vi "EVS Main Dev.vi"() -> ()   [LabVIEW 2009]
uses:
  <vilib>/userDefined/High Color/IMAQdx.ctl
  UDP Lib/UDP Network Location.ctl
  <vilib>/vision/driver/IMAQdx.llb/IMAQdx Acquisition Mode.ctl
  <vilib>/Platform/TimedLoop/XDataNode/XDataNode.xnode
  <vilib>/Platform/TimedLoop/XDataNode/loadlvalarms.vi
  <vilib>/Platform/TimedLoop/XDataNode/timing_clust.ctl
  <vilib>/Platform/TimedLoop/XDataNode/nitl_modes.ctl
  <vilib>/Platform/TimedLoop/XDataNode/wakeup.ctl
  <vilib>/vision/driver/NI_Vision_Acquisition_Software.lvlib
  <vilib>/Platform/TimedLoop/XDataNode/XDNodeRunTimeDep.lvlib
panel:
  out "Extracted 2":T1(plugin-control) caption="Extracted"
  in  "IMAQdx Session Center":T2="rcam" caption="Center Session"
  out "Original":T1(plugin-control)
  out "Extracted":T1(plugin-control)
  out "Ramp?":bool
  out "Iteration Duration":i64
  out "Number of ramp regions (left)":i32
  out "Number of ramp regions (right)":i32
  out "Sick array":u16[](array[numeric])
  in  "stop":bool
  out "HB":bool
  in  "IMAQdx Session Left":T2="lcam" caption="Left Session"
  in  "IMAQdx Session Right":T2="rcam" caption="Right Session"
  # "0: Original\n1: Extracted\n2: Masked"
  # "0: Old line extraction\n1: Solid white line (ramp)\n2: LPF"
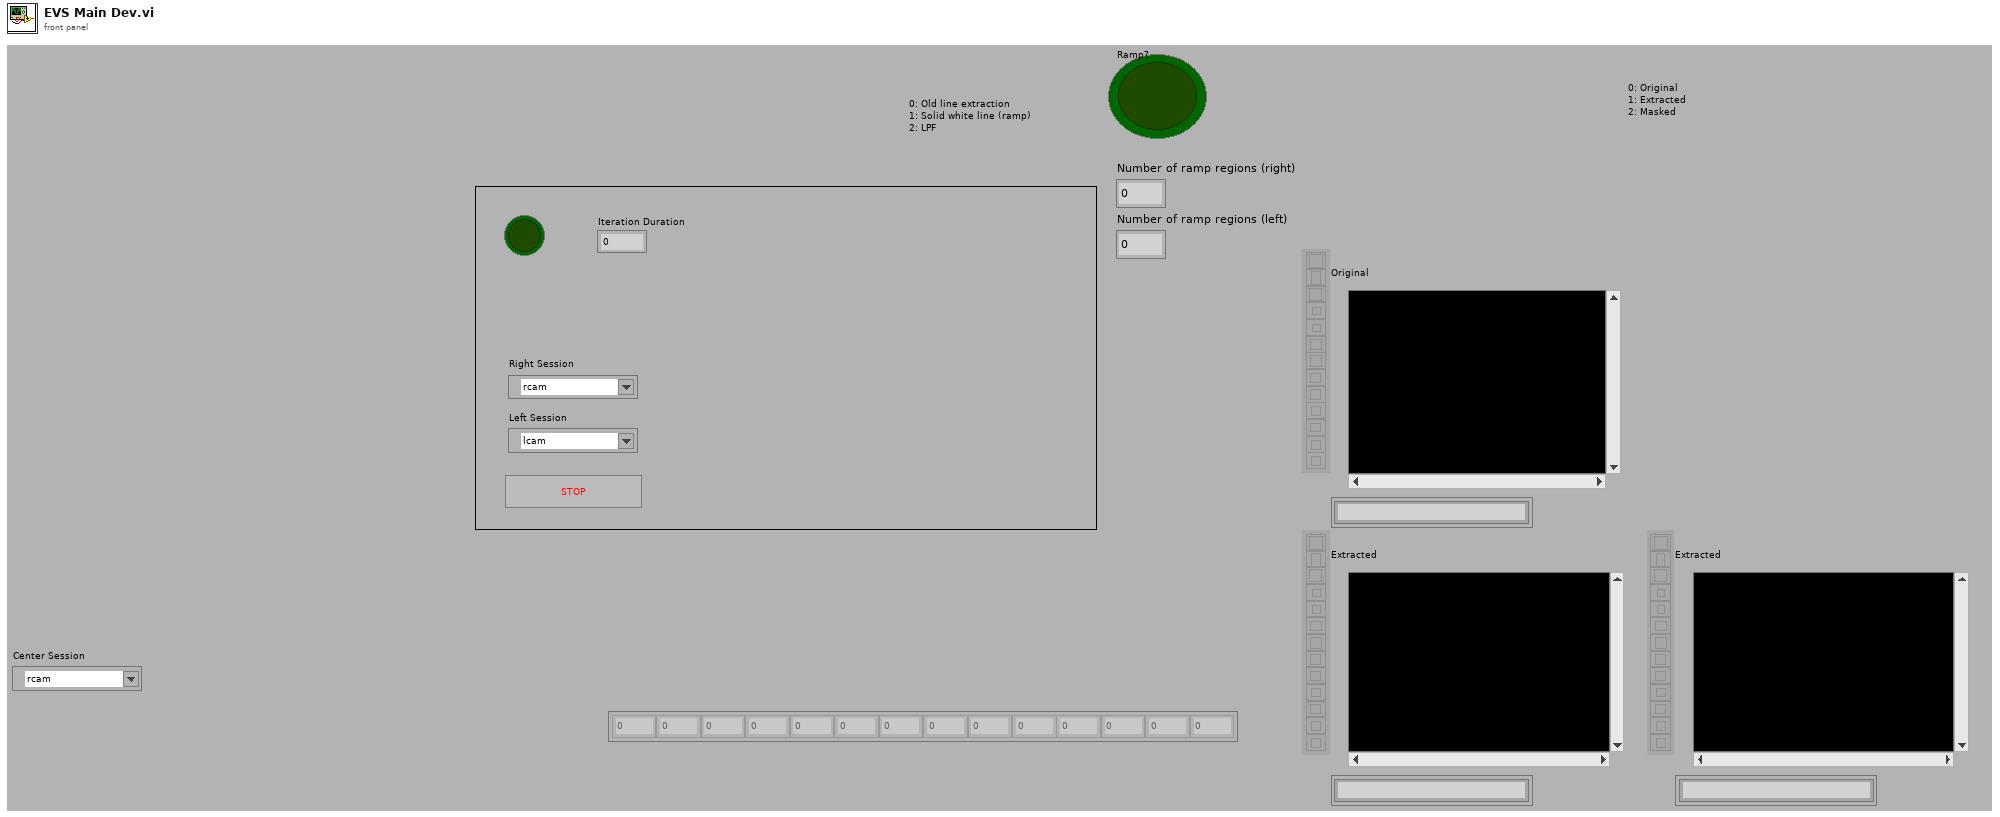
[diagram p1: front panel]
types:
  T1 = typedef "IMAQ Image.ctl" = refnum<image>
  T2 = typedef "IMAQdx.ctl" = refnum<k21>
  T3 = cluster{"Sick array":u16[], "Camera init":bool, "Objects Array":cluster{"X Coord":dbl[], "Y Coord":dbl[]}[]}
  T4 = typedef "NI_Vision_Acquisition_Software.lvlib/IMAQdx Acquisition Mode.ctl" = enum32{"One Shot", "Continuous"}
  T5 = typedef "XDNodeRunTimeDep.lvlib/timing_clust.ctl" = cluster{"Expected End [f-1]":u64, "Actual End [f-1]":u64, "Finished Late? [f-1]":bool, "Expected End [i-1]":u64, "Actual End [i-1]":u64, "Finished Late? [i-1]":bool, "Expected Start [i]":u64, "Actual Start [i]":u64, "Expected Start [f]":u64, "Actual Start [f]":u64, "Source Name":string, "Structure Name":string, "Period":i64, "Deadline":i64, "Offset":i64, "Start":i64, "Priority":i32, "Timeout":i32, "Mode":T6, "Wakeup Reason":T7, "Error":errorcluster, "Source Type":string, "Secondary Source Type":string, "Global End Time":u64, "Global Start Time":u64, "Frame Duration":u64, "Iteration Duration":u64, "Assigned CPU":i32, "I/O Scan Engine Mode":u32}
  T6 = typedef "XDNodeRunTimeDep.lvlib/nitl_modes.ctl" = enum32{"No Change", "Process missed periods, maintain original phase", "Discard missed periods, maintain original phase", "Process missed periods, ignore original phase", "Discard missed periods, ignore original phase"}
  T7 = typedef "XDNodeRunTimeDep.lvlib/wakeup.ctl" = enum32{"Normal", "Aborted", "Asynchronous wakeup", "Timing source error", "Timed loop error", "Timeout"}
  T8 = typedef "UDP Network Location.ctl" = cluster{"IP Address":string, "Port":u16}
  T9 = typedef "UDP Base.ctl" = cluster{"UDP Session":refnum<k16>, "UDP Socket Params":T10}
  T10 = typedef "UDP Socket Params.ctl" = cluster{"Local Port":u16, "Read Timeout":i32, "Write Timeout":i32}
  T11 = typedef "Image Type" = u32
  T12 = cluster{"Sick array":u16[], "Camera init":bool, "Objects Array":cluster{"X Coord":dbl[], "Y Coord":dbl[]}[], bool}
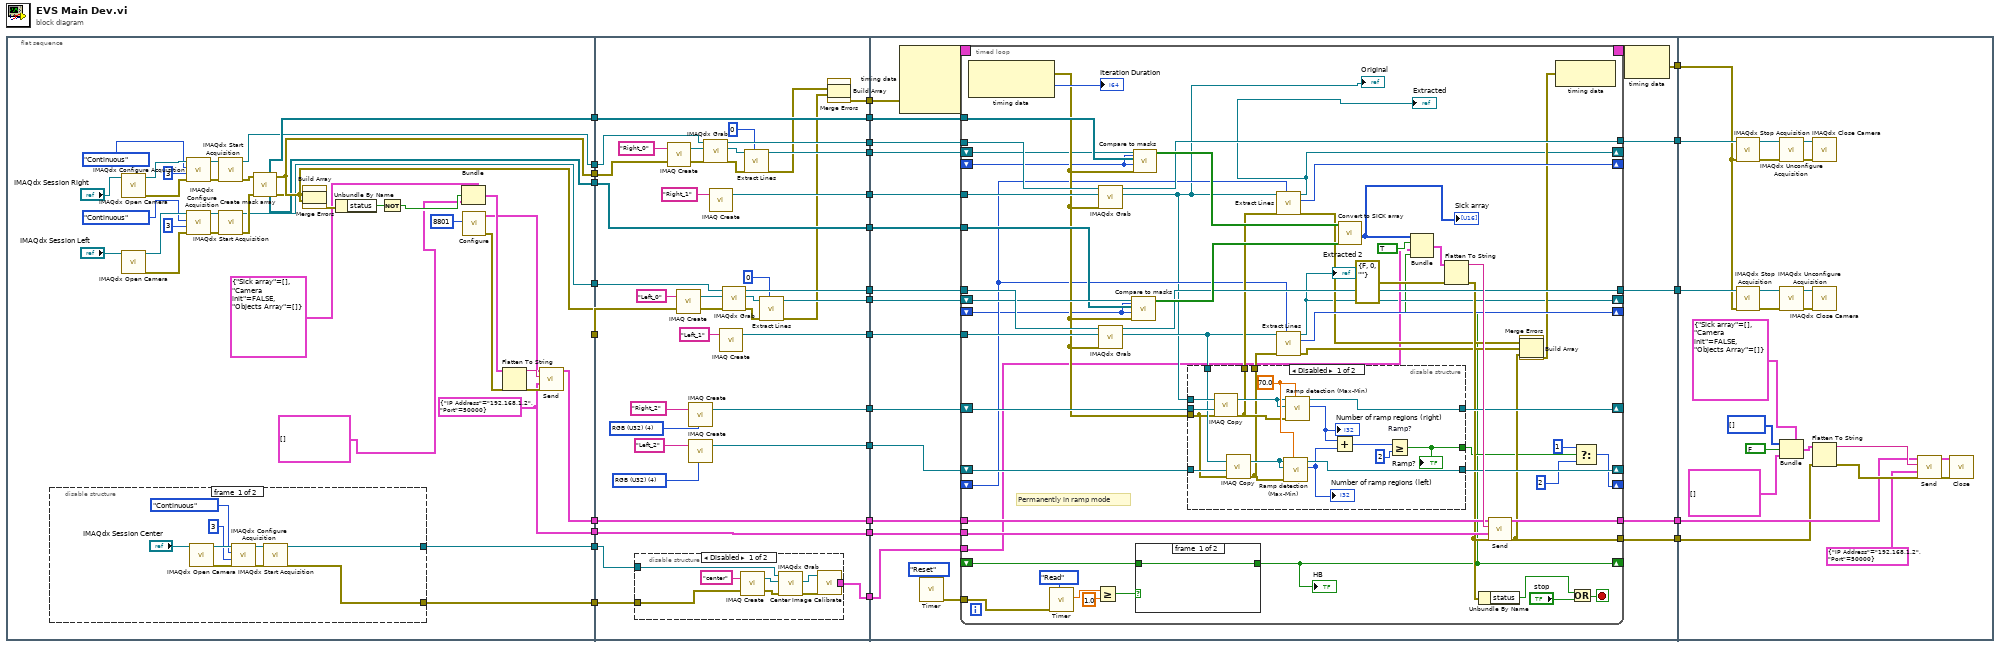
[diagram p0: block diagram]
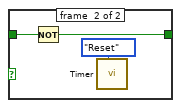
[diagram p4: hidden frame]
diagram:
  n1 = flat-sequence {
    tunnel: [w47] -> w29
    tunnel: [w46] -> w28
    tunnel: [w45] -> w27
    tunnel: [w35] -> w26
    tunnel: [w44] -> w19
    tunnel: [w43] -> w17
    tunnel: [w42] -> w16
    tunnel: [w39] -> w8
    tunnel: [w34] -> w3
    tunnel: [w33] -> w2
    tunnel: w29 -> [w109]
    tunnel: w28 -> [w108]
    tunnel: w27 -> [w105]
    tunnel: w26 -> [w104]
    tunnel: [w103] -> w25
    tunnel: [w100] -> w24
    tunnel: [w99] -> w23
    tunnel: [w98] -> w22
    tunnel: [w97] -> w21
    tunnel: [w96] -> w20
    tunnel: w19 -> [w95]
    tunnel: [w95] -> w18
    tunnel: w17 -> [w94]
    tunnel: w16 -> [w93]
    tunnel: [w94] -> w15
    tunnel: [w93] -> w14
    tunnel: [w92] -> w9
    tunnel: w8 -> [w92]
    tunnel: [w89] -> w7
    tunnel: [w88] -> w6
    tunnel: [w85] -> w5
    tunnel: w3 -> [w80]
    tunnel: w2 -> [w79]
    tunnel: [w78] -> w1
    tunnel: w25 -> [w137]
    tunnel: w24 -> [w136]
    tunnel: w23 -> [w148]
    tunnel: w22 -> [w147]
    tunnel: w21 -> [w146]
    tunnel: w20 -> [w145]
    tunnel: w18 -> [w144]
    tunnel: w15 -> [w143]
    tunnel: w14 -> [w142]
    tunnel: [w141] -> w13
    tunnel: [w140] -> w12
    tunnel: [w139] -> w11
    tunnel: [w138] -> w10
    tunnel: w9 -> [w135]
    tunnel: w7 -> [w132]
    tunnel: w6 -> [w131]
    tunnel: w5 -> [w130]
    tunnel: [w129] -> w4
    tunnel: w1 -> [w128]
    tunnel: w13 -> [w253]
    tunnel: w12 -> [w252]
    tunnel: w11 -> [w248]
    tunnel: w10 -> [w247]
    tunnel: w4 -> [w241]
    frame #0 {
      w39 = T8 {"IP Address"="192.168.1.2", "Port"=50000} ("cRIO Network Location")
      n2 = disable-structure shown="Enabled" {
        disable-tunnel: [w69 _] -> w34
        disable-tunnel: [w68 _] -> w33
        frame #0 {
          n3 = call <vilib>:"IMAQdx Open Camera.vi"("Session In"="IMAQdx Session Center") -> ("error out"=w75:errorcluster, "Session Out"=w74:T2)  [unwired: 2 in, 7 out]
          n4 = call <vilib>:"IMAQdx Configure Acquisition.vi"("error in"=w75, "Number of Buffers"=u32 3, "Continuous?"=IMAQdx_Acquisition_Mode."Continuous", "Session In"=w74) -> ("error out"=w76:errorcluster, "Session Out"=w73:T2)  [unwired: 1 in, 5 out]
          n5 = call <vilib>:"IMAQdx Start Acquisition.vi"("error in"=w76, "Session In"=w73) -> ("error out"=w68:errorcluster, "Session Out"=w69:T2)  [unwired: 8 out]
        }
        frame #1 {
        }
      }
      n6 = call <vilib>:"IMAQdx Open Camera.vi"("Session In"="IMAQdx Session Right") -> ("error out"=w66:errorcluster, "Session Out"=w65:T2)  [unwired: 2 in, 7 out]
      n7 = call <vilib>:"IMAQdx Open Camera.vi"("Session In"="IMAQdx Session Left") -> ("error out"=w60:errorcluster, "Session Out"=w61:T2)  [unwired: 2 in, 7 out]
      n8 = call <vilib>:"IMAQdx Configure Acquisition.vi"("error in"=w66, "Number of Buffers"=u32 3, "Continuous?"=IMAQdx_Acquisition_Mode."Continuous", "Session In"=w65) -> ("error out"=w67:errorcluster, "Session Out"=w64:T2)  [unwired: 1 in, 5 out]
      n9 = call <vilib>:"IMAQdx Configure Acquisition.vi"("error in"=w60, "Number of Buffers"=u32 3, "Continuous?"=IMAQdx_Acquisition_Mode."Continuous", "Session In"=w61) -> ("error out"=w59:errorcluster, "Session Out"=w62:T2)  [unwired: 1 in, 5 out]
      n10 = call <vilib>:"IMAQdx Start Acquisition.vi"("error in"=w67, "Session In"=w64) -> ("error out"=w53:errorcluster, "Session Out"=w35:T2)  [unwired: 8 out]
      n11 = call <vilib>:"IMAQdx Start Acquisition.vi"("error in"=w59, "Session In"=w62) -> ("error out"=w52:errorcluster, "Session Out"=w45:T2)  [unwired: 8 out]
      n12 = call "Create mask array.vi"("Left error in"=w52, "Right Error in"=w53) -> ("Left error out"=w46:errorcluster, "Right error out"=w47:errorcluster, "Left Cam Masks"=w42:T1[], "Right Cam Masks"=w43:T1[])  [unwired: 6 in]
      n13 = Build Array(w47, w46) -> (w32:errorcluster[])
      n14 = call <vilib>:"Merge Errors.vi"("error array in"=w32) -> ("error out"=w40:errorcluster)  [unwired: 6 in]
      n15 = Unbundle By Name(w40) -> ("status"=w51:bool)
      n16 = Not(x=w51) -> (.not. x?=w41:bool)
      n17 = Bundle(cluster=T3 {"Sick array"=[], "Camera init"=FALSE, "Objects Array"=[]}, "Camera init"=w41, "Objects Array"=cluster{"X Coord":dbl[], "Y Coord":dbl[]}[] []) -> (w50:T3)  [unwired: 1 in]
      n18 = call "Configure.vi"("Local Port"=u16 8801) -> ("error out"=w36:errorcluster, "UDP Base out"=w37:T9)  [unwired: 9 in]
      n19 = Flatten To String(anything=w50, error in (no error)=w36) -> (data string=w49:string, error out=w48:errorcluster)  [unwired: 2 in, 1 out]
      n20 = call "Send.vi"("error in (no error)"=w48, "Destination Location"=w39, "Send Data"=w49, "UDP Base in"=w37) -> ("UDP Base out"=w44:T9)  [unwired: 5 in, 2 out]
    }
    frame #1 {
      w83 = T11 4 items=["Grayscale (U8)", "Grayscale (I16)", "Grayscale (SGL)", "Complex (CSG)", "RGB (U32)", "HSL (U32)", "RGB (U64)", "Grayscale (U16)"] ("Image Type")
      w84 = T11 4 items=["Grayscale (U8)", "Grayscale (I16)", "Grayscale (SGL)", "Complex (CSG)", "RGB (U32)", "HSL (U32)", "RGB (U64)", "Grayscale (U16)"] ("Image Type")
      n21 = disable-structure shown="Disabled" {
        disable-tunnel: w80 -> [w120 _]
        disable-tunnel: w79 -> [w119 _]
        disable-tunnel: [w118 _] -> w78
        frame #0 {
          n22 = call "IMAQ Create"("Image Name"="center", "error in (no error)"=w119) -> ("New Image"=w121:T1, "error out"=w122:errorcluster)  [unwired: 3 in]
          n23 = call <vilib>:"IMAQdx Grab.vi"("error in"=w122, "Image In"=w121, "Session In"=w120) -> ("error out"=w125:errorcluster, "Image Out"=w124:T1)  [unwired: 5 in, 2 out]
          n24 = call "Center Image Calibrate.vi"("error in"=w125, "Image In"=w124) -> ("Objects Array"=w118:cluster{"X Coord":dbl[], "Y Coord":dbl[]}[])  [unwired: 1 in, 2 out]
        }
        frame #1 {
        }
      }
      n25 = call "IMAQ Create"("Image Name"="Right_0", "error in (no error)"=w109) -> ("New Image"=w111:T1, "error out"=w110:errorcluster)  [unwired: 3 in]
      n26 = call "IMAQ Create"("Image Name"="Left_0", "error in (no error)"=w108) -> ("New Image"=w113:T1, "error out"=w112:errorcluster)  [unwired: 3 in]
      n27 = call "IMAQ Create"("Image Name"="Right_2", "Image Type"=w84) -> ("New Image"=w89:T1)  [unwired: 3 in, 1 out]
      n28 = call "IMAQ Create"("Image Name"="Left_2", "Image Type"=w83) -> ("New Image"=w88:T1)  [unwired: 3 in, 1 out]
      n29 = call <vilib>:"IMAQdx Grab.vi"("error in"=w110, "Image In"=w111, "Session In"=w104) -> ("error out"=w117:errorcluster, "Image Out"=w114:T1, "Session Out"=w99:T2)  [unwired: 5 in, 1 out]
      n30 = call "IMAQ Create"("Image Name"="Right_1") -> ("New Image"=w103:T1)  [unwired: 4 in, 1 out]
      n31 = call "IMAQ Create"("Image Name"="Left_1") -> ("New Image"=w100:T1)  [unwired: 4 in, 1 out]
      n32 = call <vilib>:"IMAQdx Grab.vi"("error in"=w112, "Image In"=w113, "Session In"=w105) -> ("error out"=w116:errorcluster, "Image Out"=w115:T1, "Session Out"=w98:T2)  [unwired: 5 in, 1 out]
      n33 = call "Extract Lines.vi"("Extraction mode"=0, "error in (no error)"=w117, "Image Src"=w114) -> ("error out"=w87:errorcluster, "Image Out"=w97:T1)  [unwired: 6 in, 1 out]
      n34 = call "Extract Lines.vi"("Extraction mode"=0, "error in (no error)"=w116, "Image Src"=w115) -> ("error out"=w86:errorcluster, "Image Out"=w96:T1)  [unwired: 6 in, 1 out]
      n35 = Build Array(w87, w86) -> (w77:errorcluster[])
      n36 = call <vilib>:"Merge Errors.vi"("error array in"=w77) -> ("error out"=w85:errorcluster)  [unwired: 6 in]
    }
    frame #2 {
      n37 = node-c288(w130) -> (w134:T5)  [unwired: 3 in]
      n38 = call "Timer.vi"("Cmd"=enum16{"Reset", "Read"}."Reset") -> ("error out"=w126:errorcluster)  [unwired: 9 in, 1 out]
      n39 = timed-loop {
        tunnel: w148 -> [w206]
        tunnel: w147 -> [w205]
        shift-right: [w161] -> _
        shift-left: w146 -> [w162]
        shift-right: [w155] -> _
        shift-left: w145 -> [w204]
        shift-right: [w179] -> _
        shift-left: _ -> [w158]
        shift-right: [w180] -> _
        shift-left: _ -> [w159]
        tunnel: w144 -> [w200]
        tunnel: [w199] -> w139
        tunnel: [w173] -> w138
        tunnel: w143 -> [w198]
        tunnel: w142 -> [w197]
        tunnel: [w196] -> w140
        tunnel: [w195] -> w141
        tunnel: w137 -> [w194]
        tunnel: w136 -> [w193]
        tunnel: w135 -> [w189]
        shift-right: [w149] -> _
        shift-left: _ -> [w188]
        timing: w134 -> [_]
        timing-out: [_] -> w133
        shift-right: [w186] -> _
        shift-left: w132 -> [w178]
        shift-right: [w185] -> _
        shift-left: w131 -> [w177]
        shift-right: [w164] -> _
        shift-left: _ -> [w168]
        tunnel: w128 -> [w157]
        tunnel: w126 -> [w153]
        stop <- w184 stop-if-true
        # "Permanently in ramp mode"
        n40 = node-c288() -> (w176:errorcluster, →"Iteration Duration":i64)  [unwired: 1 in]
        n41 = call "Timer.vi"("Cmd"=enum16{"Reset", "Read"}."Read", "error in (no error)"=w153) -> ("Elapsed Time"=w152:dbl)  [unwired: 8 in, 1 out]
        n42 = Greater Or Equal?(x=w152, y=1.0) -> (x >= y?=w150:bool)
        n43 = call <vilib>:"IMAQdx Grab.vi"("error in"=w176, "Image In"=w194, "Session In"=w206) -> ("Image Out"=w160:T1, "Session Out"=w196:T2)  [unwired: 5 in, 2 out]
        "Original" <- w160
        n44 = call <vilib>:"IMAQdx Grab.vi"("error in"=w176, "Image In"=w193, "Session In"=w205) -> ("Image Out"=w163:T1, "Session Out"=w195:T2)  [unwired: 5 in, 2 out]
        n45 = call "Compare to masks.vi"("Number of Particles1"=w158, "error in (no error)"=w176, "Number of Particles"=w158, "Mask array"=w197, "Image Src"=w204) -> ("Marked Regions"=w202:bool[])  [unwired: 5 in, 1 out]
        n46 = call "Compare to masks.vi"("Number of Particles1"=w159, "error in (no error)"=w176, "Number of Particles"=w159, "Mask array"=w198, "Image Src"=w162) -> ("Marked Regions"=w203:bool[])  [unwired: 5 in, 1 out]
        n47 = case shown="True" w150 {
          tunnel: [w207 w210] -> w149
          tunnel: w188 -> [w207 w209]
          frame #0 {
          }
          frame #1 {
            n48 = Not(x=w209) -> (.not. x?=w210:bool)
            n49 = call "Timer.vi"("Cmd"=enum16{"Reset", "Read"}."Reset") -> ()  [unwired: 9 in, 2 out]
          }
        }
        "HB" <- w149
        n50 = disable-structure shown="Disabled" {
          disable-tunnel: [w227 _] -> w186
          disable-tunnel: [w226 _] -> w185
          disable-tunnel: [w220 _] -> w167
          disable-tunnel: w178 -> [w219 _]
          disable-tunnel: w160 -> [w218 _]
          disable-tunnel: w163 -> [w217 _]
          disable-tunnel: w177 -> [w216 _]
          disable-tunnel: w176 -> [w215 _]
          disable-tunnel: [w212 _] -> w170
          disable-tunnel: [w211 _] -> w169
          frame #0 {
            w225 = sgl 70.0 ("Tolerance")
            n51 = call "IMAQ Copy"("error in (no error)"=w215, "Image Dst"=w219, "Image Src"=w218) -> ("error out"=w212:errorcluster, "Image Dst Out"=w214:T1)  [unwired: 3 in]
            n52 = call "IMAQ Copy"("error in (no error)"=w215, "Image Dst"=w216, "Image Src"=w217) -> ("error out"=w211:errorcluster, "Image Dst Out"=w213:T1)  [unwired: 3 in]
            n53 = call "Ramp detection (Max-Min).vi"("Tolerance"=w225, "error in (no error)"=w211, "Image Dst"=w213, "Image Src"=w213) -> ("Number of ramp regions"=w223:i32, "Image Out"=w226:T1)  [unwired: 5 in, 1 out]
            "Number of ramp regions (left)" <- w223
            n54 = call "Ramp detection (Max-Min).vi"("Tolerance"=w225, "error in (no error)"=w212, "Image Dst"=w214, "Image Src"=w214) -> ("Number of ramp regions"=w224:i32, "Image Out"=w227:T1)  [unwired: 5 in, 1 out]
            "Number of ramp regions (right)" <- w224
            n55 = Add(x=w224, y=w223) -> (x+y=w222:i32)
            n56 = Greater Or Equal? "Ramp?"(x=w222, y=2) -> (x >= y?=w220:bool)
            "Ramp?" <- w220
          }
          frame #1 {
          }
        }
        n57 = call "Extract Lines.vi"("Extraction mode"=w168, "error in (no error)"=w170, "Image Src"=w160) -> ("error out"=w172:errorcluster, "Number of Particles1"=w180:i32, "Image Out"=w161:T1)  [unwired: 6 in]
        "Extracted" <- w161
        n58 = call "Extract Lines.vi"("Extraction mode"=w168, "error in (no error)"=w169, "Image Src"=w163) -> ("error out"=w171:errorcluster, "Number of Particles1"=w179:i32, "Image Out"=w155:T1)  [unwired: 6 in]
        "Extracted 2" <- w155
        n59 = call "Convert to SICK array.vi"("Left Regions"=w202, "Right Regions"=w203) -> ("Sick array"=w175:u16[])  [unwired: 9 in]
        "Sick array" <- w175
        n60 = Bundle("Sick array"=w175, "Camera init"=TRUE, "Objects Array"=w157, w149) -> (w190:T12)  [unwired: 1 in]
        n61 = Flatten To String(anything=w190, error in (no error)=errorcluster {"status"=FALSE, "code"=0, "source"=""} ("error out")) -> (data string=w201:string, error out=w181:errorcluster)  [unwired: 2 in, 1 out]
        n62 = Unbundle By Name(w181) -> ("status"=w192:bool)
        n63 = call "Send.vi"("error in (no error)"=w181, "Destination Location"=w189, "Send Data"=w201, "UDP Base in"=w200) -> ("error out"=w173:errorcluster, "UDP Base out"=w199:T9)  [unwired: 5 in, 1 out]
        n64 = Build Array(w172, w171, w173) -> (w156:errorcluster[])
        n65 = call <vilib>:"Merge Errors.vi"("error array in"=w156) -> ("error out"=w174:errorcluster)  [unwired: 6 in]
        n66 = node-c288(w174) -> ()  [unwired: 1 out]
        n67 = Or(x=w192, y="stop") -> (x .or. y?=w184:bool)
        n68 = Select(t=1, s=w167, f=2 ("Extraction mode")) -> (s? t:f=w164:i32)
      }
      n69 = node-c288(w133) -> (w129:errorcluster)
    }
    frame #3 {
      n70 = call <vilib>:"IMAQdx Stop Acquisition.vi"("error in"=w241, "Session In"=w252) -> ("error out"=w259:errorcluster, "Session Out"=w258:T2)  [unwired: 8 out]
      n71 = call <vilib>:"IMAQdx Stop Acquisition.vi"("error in"=w241, "Session In"=w253) -> ("error out"=w255:errorcluster, "Session Out"=w254:T2)  [unwired: 8 out]
      n72 = call <vilib>:"IMAQdx Unconfigure Acquisition.vi"("error in"=w259, "Session In"=w258) -> ("error out"=w260:errorcluster, "Session Out"=w261:T2)  [unwired: 8 out]
      n73 = call <vilib>:"IMAQdx Unconfigure Acquisition.vi"("error in"=w255, "Session In"=w254) -> ("error out"=w256:errorcluster, "Session Out"=w257:T2)  [unwired: 8 out]
      n74 = Bundle(cluster=T3 {"Sick array"=[], "Camera init"=FALSE, "Objects Array"=[]}, "Sick array"=u16[] [] ("Camera SICK"), "Camera init"=FALSE, "Objects Array"=cluster{"X Coord":dbl[], "Y Coord":dbl[]}[] []) -> (w243:T3)
      n75 = call <vilib>:"IMAQdx Close Camera.vi"("error in"=w260, "Session In"=w261) -> ()  [unwired: 10 out]
      n76 = call <vilib>:"IMAQdx Close Camera.vi"("error in"=w256, "Session In"=w257) -> ()  [unwired: 10 out]
      n77 = Flatten To String(anything=w243, error in (no error)=w247) -> (data string=w251:string, error out=w250:errorcluster)  [unwired: 2 in, 1 out]
      n78 = call "Send.vi"("error in (no error)"=w250, "Destination Location"=T8 {"IP Address"="192.168.1.2", "Port"=50000}, "Send Data"=w251, "UDP Base in"=w248) -> ("error out"=w245:errorcluster, "UDP Base out"=w246:T9)  [unwired: 5 in, 1 out]
      n79 = call "Close.vi"("error in (no error)"=w245, "Cluster of class private data"=w246) -> ()  [unwired: 9 in, 1 out]
    }
  }
